vi "test_output.vi"   [LabVIEW 2019]
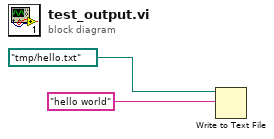
[diagram p0: block diagram]
diagram:
  n1 = Write to Text File(file (use dialog)=path "/tmp/hello.txt", text="hello world") -> ()  [unwired: 2 in, 3 out]
